vi "Load EDS.vi"(8 "error in":errorcluster, 10 "EDS File Path":path, 11 "Interactor in":refnum<class "Interactor.lvclass">) -> (0 "error out":errorcluster, 3 "Interactor out":refnum<class "Interactor.lvclass">)   [LabVIEW 2020, in "Interactor.lvlib" / "Interactor.lvclass"]
uses:
  Interactor.lvclass
  Interactor.lvclass/Interactor.ctl
  Object Dictionary UI Messages/Populate OD Msg/Populate OD Msg.lvclass
  Home Messages/EDS File Loaded Msg/EDS File Loaded Msg.lvclass
  EDS-File-Viewer/source/Electronic Datasheet/Electronic Datasheet.lvclass
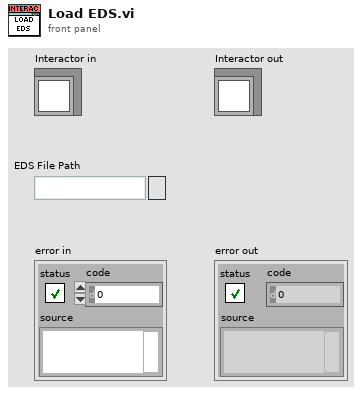
[diagram p1: front panel]
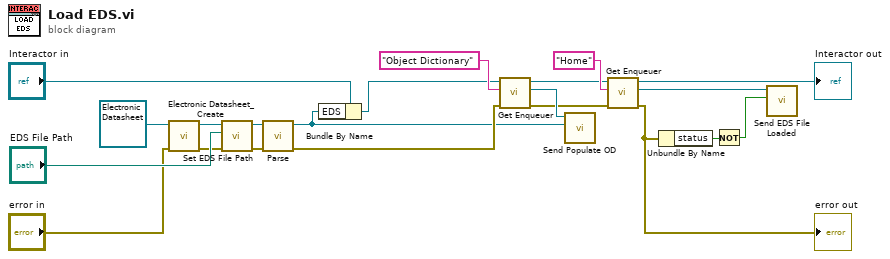
[diagram p0: block diagram]
diagram:
  n1 = call "Electronic Datasheet_Create.vi"("Error In"="error in", "reference in"=refnum<class "Electronic Datasheet.lvclass"> refnum ("EDS in")) -> ("Error Out"=w7:errorcluster, "reference out"=w8:refnum<class "Electronic Datasheet.lvclass">)  [unwired: 8 in]
  n2 = call "Set EDS File Path.vi"("error in"=w7, "EDS File Path"="EDS File Path", "reference in"=w8) -> ("error out"=w5:errorcluster, "reference out"=w20:refnum<class "Electronic Datasheet.lvclass">)  [unwired: 7 in]
  n3 = call "Parse.vi"("error in"=w5, "reference in"=w20) -> ("error out"=w12:errorcluster, "reference out"=w3:refnum<class "Electronic Datasheet.lvclass">)  [unwired: 8 in]
  n4 = Bundle By Name(cluster="Interactor in", "EDS"=w3) -> (w16:refnum<class "Interactor.lvclass">)
  n5 = call "Get Enqueuer.vi"("error in"=w12, "Ident"="Object Dictionary", "Interactor in"=w16) -> ("error out"=w1:errorcluster, "Enq"=w18:refnum<class "Message Enqueuer.lvclass">, "Interactor out"=w2:refnum<class "Interactor.lvclass">)  [unwired: 6 in]
  n6 = call "Send Populate OD.vi"("EDS"=w3, "Message Enqueuer"=w18) -> ()  [unwired: 8 in, 2 out]
  n7 = call "Get Enqueuer.vi"("error in"=w1, "Ident"="Home", "Interactor in"=w2) -> ("error out"=w4:errorcluster, "Enq"=w13:refnum<class "Message Enqueuer.lvclass">, "Interactor out"=→"Interactor out":refnum<class "Interactor.lvclass">)  [unwired: 6 in]
  "error out" <- w4
  n8 = Unbundle By Name(w4) -> ("status"=w11:bool)
  n9 = Not(x=w11) -> (.not. x?=w10:bool)
  n10 = call "Send EDS File Loaded.vi"("Valid?"=w10, "Message Enqueuer"=w13) -> ()  [unwired: 8 in, 2 out]
